vi "CRYSet Login Front Panel.vi"(11 "Vi Ref in":refnum<vi> caption="Vi Ref") -> (3 "Vi Ref out":refnum<vi> caption="Vi Ref")   [LabVIEW 2013]
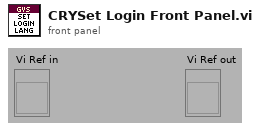
[diagram p1: front panel]
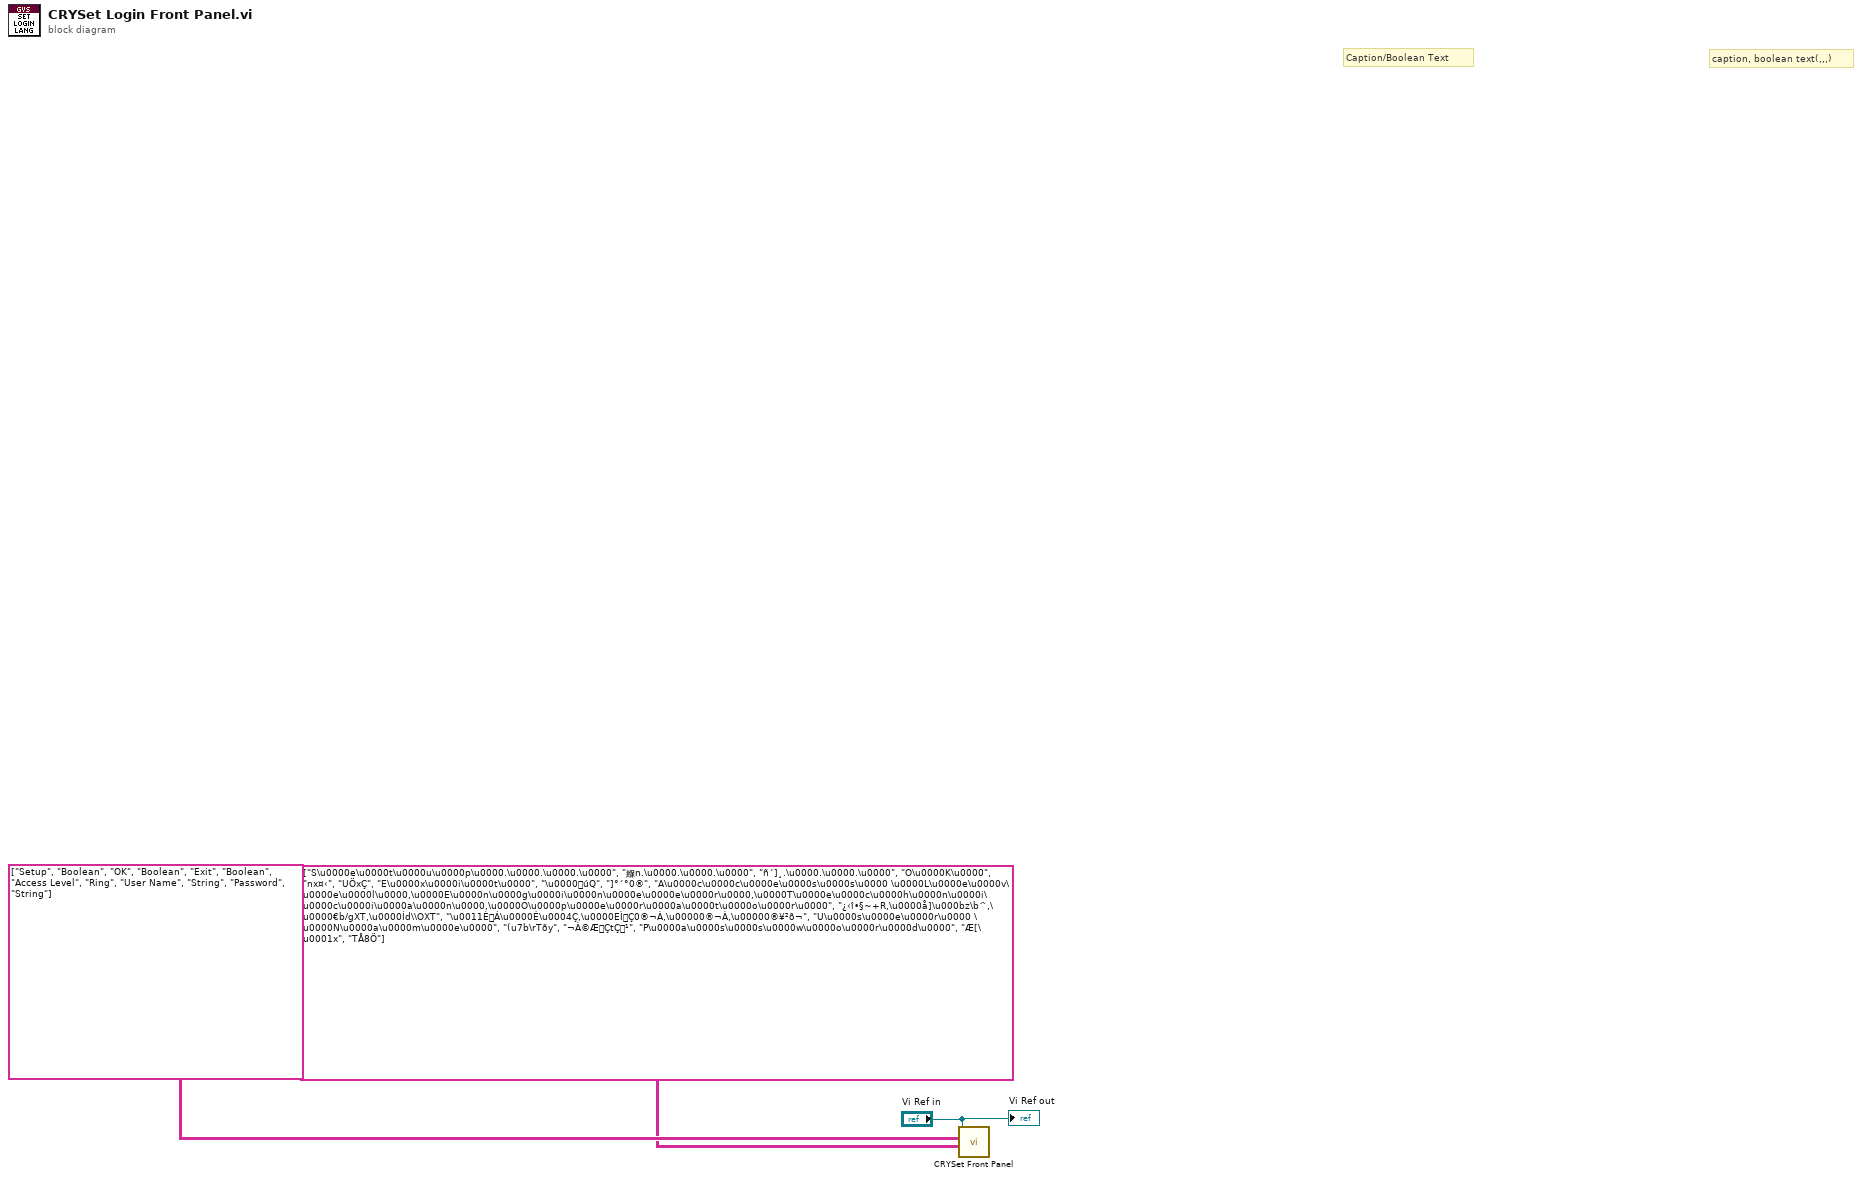
[diagram p0: block diagram]
diagram:
  # "caption, boolean text(,,,)"
  # "Caption/Boolean Text"
  n1 = call "CRYSet Front Panel.vi"("Caption(Boolean Text)"=string[][] [["S\u0000e\u0000t\u0000u\u0000p\u0000.\u0000.\u0000.\u0000", "緥n.\u0000.\u0000.\u0000", "ñ´]¸.\u0000.\u0000.\u0000"], ["O\u0000K\u0000", "nx¤‹", "UÖxÇ"], ["E\u0000x\u0000i\u0000t\u0000", "\u0000úQ", "]°´°0®"], ["A\u0000c\u0000c\u0000e\u0000s\u0000s\u0000 \u0000L\u0000e\u0000v\u0000e\u0000l\u0000,\u0000E\u0000n\u0000g\u0000i\u0000n\u0000e\u0000e\u0000r\u0000,\u0000T\u0000e\u0000c\u0000h\u0000n\u0000i\u0000c\u0000i\u0000a\u0000n\u0000,\u0000O\u0000p\u0000e\u0000r\u0000a\u0000t\u0000o\u0000r\u0000", "¿‹î•§~+R,\u0000å]\u000bz\b^,\u0000€b/gXT,\u0000Íd\\OXT", "\u0011ÈÁ\u0000É\u0004Ç,\u0000EÌÇ0®¬À,\u00000®¬À,\u00000®¥²õ¬"], ["U\u0000s\u0000e\u0000r\u0000 \u0000N\u0000a\u0000m\u0000e\u0000", "(u7b\rTðy", "¬À©ÆÇtÇ¹"], ["P\u0000a\u0000s\u0000s\u0000w\u0000o\u0000r\u0000d\u0000", "Æ[\u0001x", "TÅ8Ö"]], "Control ID and Type(Label Name, Type)"=string[][] [["Setup", "Boolean"], ["OK", "Boolean"], ["Exit", "Boolean"], ["Access Level", "Ring"], ["User Name", "String"], ["Password", "String"]], "Vi Ref"="Vi Ref in") -> ()  [unwired: 9 in]
  "Vi Ref out" <- "Vi Ref in"
